vi "WfrmToMultiPointReadingArray.vi"(8 "error in (no error)":errorcluster, 11 "data":waveform(dbl)[](array[waveform])) -> (0 "error out":errorcluster, 3 "MultiPointReadingArrayOut":T1 {"Timestamp" format="%_6f"})   [LabVIEW 2014, in "SamplerPlugins.lvlib" / "NiPxi6123.lvclass"]
uses:
  NiPxi6123.lvclass
  NISTSamplerPluginsBaseClass/TypeDefs/MultiPointReadingArrayParams.ctl
  NISTSamplerPluginsBaseClass/TypeDefs/MultiPointReadingParams.ctl
  NISTSamplerPluginsBaseClass/SamplerPluginsBase.lvclass
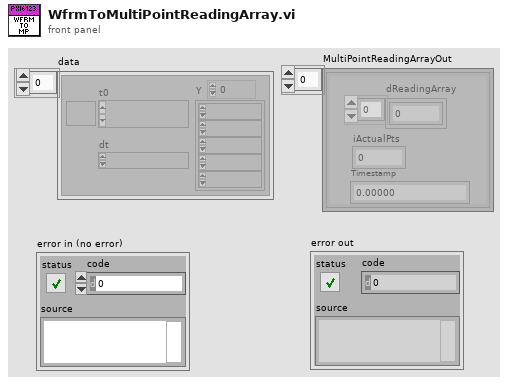
[diagram p1: front panel]
types:
  T1 = typedef "SamplerPlugins.lvlib/SamplerPluginsBase.lvclass/MultiPointReadingArrayParams.ctl" = T2[]
  T2 = typedef "SamplerPlugins.lvlib/SamplerPluginsBase.lvclass/MultiPointReadingParams.ctl" = cluster{"dReadingArray":dbl[], "iActualPts":i32, "Timestamp":dbl}
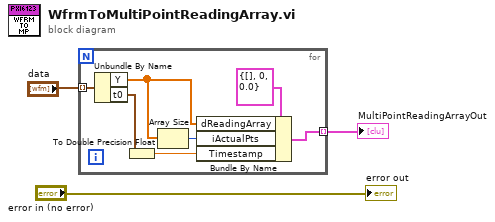
[diagram p0: block diagram]
diagram:
  n1 = for {
    tunnel: "data" -> [w7] mode=indexing
    tunnel: [w8] -> w3 mode=indexing
    n2 = Unbundle By Name(w7) -> ("Y"=w6:dbl[], "t0"=w5:timestamp)
    n3 = To Double Precision Float(number=w5) -> (double precision float=w4:dbl)
    n4 = Array Size(array=w6) -> (size(s)=w9:i32)
    n5 = Bundle By Name(cluster=T2 {"dReadingArray"=[], "iActualPts"=0, "Timestamp"=0.0} ("MultiPointReadingParams"), "dReadingArray"=w6, "iActualPts"=w9, "Timestamp"=w4) -> (w8:T2)
  }
  "MultiPointReadingArrayOut" <- w3
  "error out" <- "error in (no error)"
